vi "Device Clear.vi"(8 "error in (no error)":errorcluster, 11 "VISA Resource Name":refnum<visa-resource-name>) -> (0 "error out":errorcluster, 3 "VISA Resource Out":refnum<visa-resource-name>)   [LabVIEW 2019, in "Lake Shore 325.lvlib"]
doc: "Device clear is an IEEE-488 low-level bus message. It clears Model 325 interface activity and puts it into a bus idle state."
uses:
  <instrlib>/Lake Shore 325/Lake Shore 325.lvlib
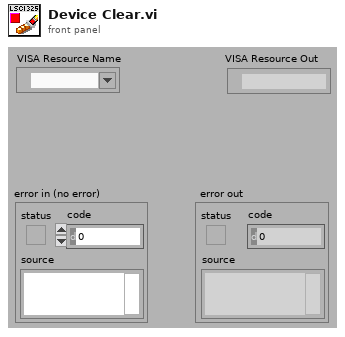
[diagram p1: front panel]
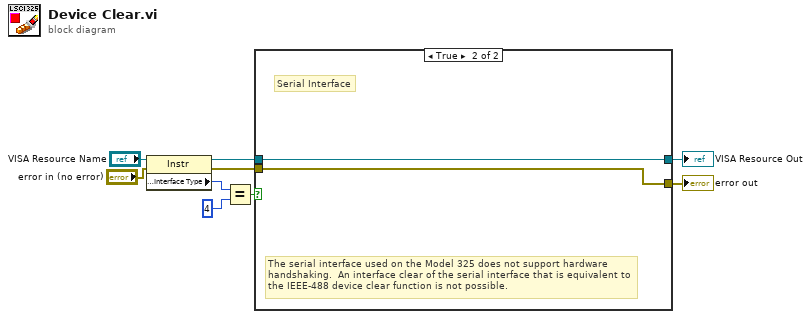
[diagram p0: block diagram]
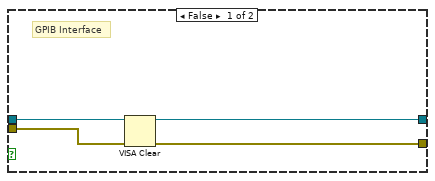
[diagram p2: hidden frame]
diagram:
  n1 = property class="Instr"(reference="VISA Resource Name", error in="error in (no error)") -> (reference out=w9:refnum<visa-resource-name>, error out=w5:errorcluster, "Interface Information:Interface Type"=w4:u16)
  n2 = Equal?(x=w4, y=u16 4) -> (x = y?=w8:bool)
  n3 = case shown="True" w8 {
    tunnel: w5 -> [w10 w15]
    tunnel: [w12 w14] -> w2
    tunnel: [w11 w15] -> w1
    tunnel: w9 -> [w13 w14]
    frame False {
      # "GPIB Interface"
      n4 = VISA Clear(VISA resource name=w13, error in (no error)=w10) -> (VISA resource name out=w12:refnum<visa-resource-name>, error out=w11:errorcluster)
    }
    frame True {
      # "The serial interface used on the Model 325 does not support hardware handshaking.  An interface clear of the serial interface that is equivalent to the IEEE-488 device clear function is not possible."
      # "Serial Interface"
    }
  }
  "VISA Resource Out" <- w2
  "error out" <- w1
